vi "PrintVI.vi"(10 "next shot":string, 11 "reference":refnum<vi>) -> ()   [LabVIEW 2013]
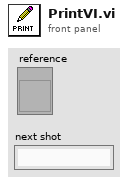
[diagram p1: front panel]
types:
  T1 = typedef "imagedata.ctl" = cluster{"image type":i32, "image depth":i32, "image":u8[], "mask":u8[], "colors":u32[], "Rectangle":cluster{"left":i16, "top":i16, "right":i16, "bottom":i16}}
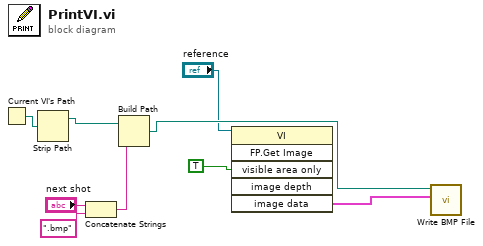
[diagram p0: block diagram]
diagram:
  n1 = Current VI's Path() -> (path=w8:path)
  n2 = Strip Path(path=w8) -> (stripped path=w9:path)  [unwired: 1 out]
  n3 = Concatenate Strings("next shot", ".bmp" ("string")) -> (w6:string)
  n4 = Build Path(base path=w9, name or relative path=w6) -> (appended path=w7:path)
  n5 = invoke class="VI" method="FP.Get Image"(reference="reference", "visible area only"=TRUE ("Nur sichtbarer Bereich")) -> ("image data"=w4:T1)  [unwired: 4 in, 5 out]
  n6 = call <vilib>:"Write BMP File.vi"("image data"=w4, "path to BMP file"=w7) -> ()  [unwired: 8 in, 2 out]
